vi "Pre Launch Init.vi"(11 "Iterator Actor in":refnum<class "Abstract Iterator Actor.lvclass">) -> (0 "error out":errorcluster, 3 "Iterator Actor out":refnum<class "Abstract Iterator Actor.lvclass">)   [LabVIEW 2023, in "Iterator Actor.lvlib" / "Abstract Iterator Actor.lvclass"]
doc: "(<B>Filename</B>: Actor Framework.lvlib:Actor.lvclass:Pre Launch Init.vi)\n\nDefines behavior that occurs after the Launch Nested Actor method is invoked but before the actor's Actor Core method begins running.\n\nBy default, this method does nothing. A descendant class may override it to define behavior."
uses:
  Abstract Iterator Actor.lvclass
  Abstract Iterator Actor.lvclass/Abstract Iterator Actor.ctl
  <vilib>/LS Instruments AG/Async Methods Actor/Async Methods Actor/Async Methods Actor/Async Methods Actor.lvclass
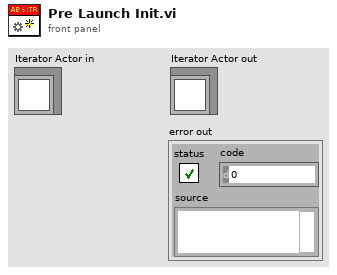
[diagram p1: front panel]
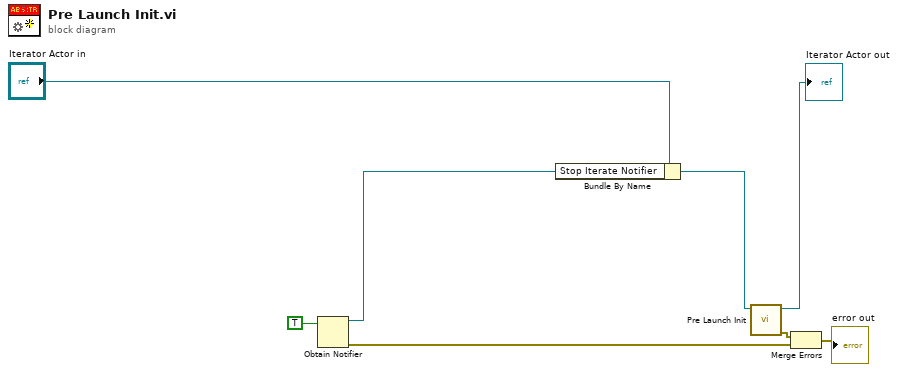
[diagram p0: block diagram]
diagram:
  n1 = Obtain Notifier(notification data type=TRUE) -> (notifier out=w7:refnum<notifier>, error out=w5:errorcluster)  [unwired: 3 in, 1 out]
  n2 = Bundle By Name(cluster="Iterator Actor in", "Stop Iterate Notifier"=w7) -> (w4:refnum<class "Abstract Iterator Actor.lvclass">)
  n3 = call-parent "Pre Launch Init.vi"("Async Methods Actor in"=w4) -> ("error out"=w1:errorcluster, "Async Methods Actor out"=→"Iterator Actor out":refnum<class "Abstract Iterator Actor.lvclass">)  [unwired: 9 in]
  n4 = Merge Errors(w1, w5) -> (→"error out":errorcluster)
